vi "TestInsertIntoPanel_OK.vi"(8 "error in (no error)":errorcluster, 11 "TestCase in":refnum<class "TestProtectedSubpanel.lvclass">) -> (0 "error out":errorcluster, 3 "TestCase out":refnum<class "TestProtectedSubpanel.lvclass">)   [LabVIEW 2015, in "TestProtectedSubpanel.lvclass"]
uses:
  TestProtectedSubpanel.lvclass
  ProtectedSubpanel.lvclass
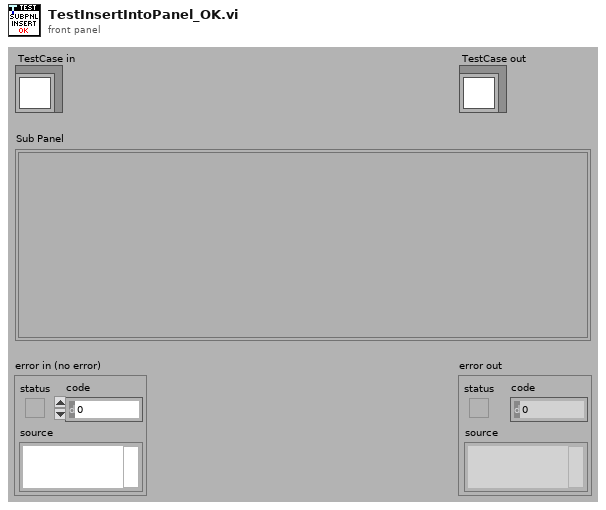
[diagram p1: front panel]
types:
  T1 = typedef "ProtectedSubpanel.lvlib/ProtectedSubpanel.lvclass/Protected Subpanel Reference.ctl" = refnum<data-value>
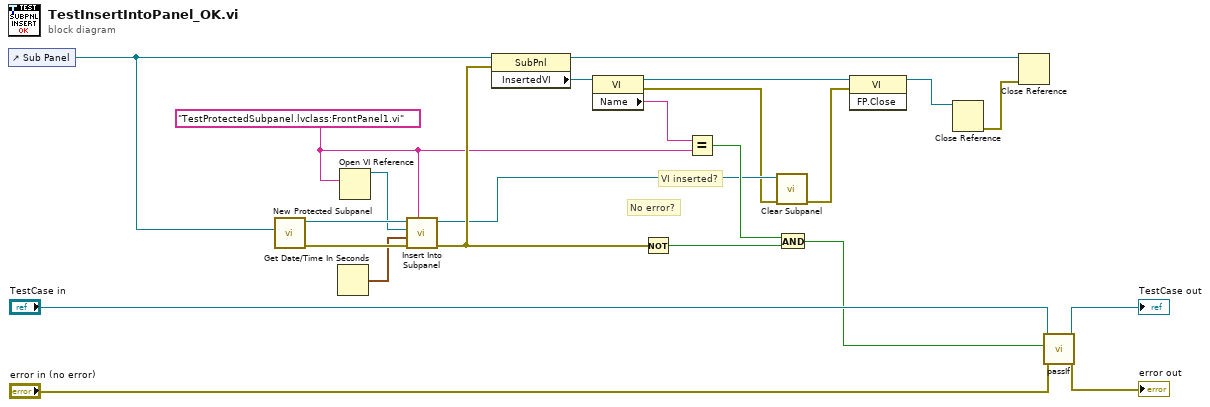
[diagram p0: block diagram]
diagram:
  w11 = "TestProtectedSubpanel.lvclass:FrontPanel1.vi"
  # "No error?"
  # "VI inserted?"
  n1 = control-ref of="Sub Panel"() -> (w17:refnum<vi>)
  n2 = call "New Protected Subpanel.vi"("SubPnl Refnum"=w17) -> ("error out"=w2:errorcluster, "Protected Subpanel"=w19:T1)  [unwired: 9 in]
  n3 = Get Date/Time In Seconds() -> (seconds since 1Jan1904=w1:timestamp)
  n4 = Open VI Reference(vi path=w11) -> (vi reference=w18:refnum<vi>)  [unwired: 5 in, 1 out]
  n5 = call "Insert Into Subpanel.vi"("Viewable Name"=w11, "error in (no error)"=w2, "Insertion Request Time"=w1, "VI Refnum"=w18, "Protected Subpanel"=w19) -> ("error out"=w14:errorcluster, "Protected Subpanel"=w5:T1)  [unwired: 5 in]
  n6 = property class="SubPnl"(reference=w17, error in=w14) -> (reference out=w9:refnum<vi>, "InsertedVI"=w13:refnum<vi>)  [unwired: 1 out]
  n7 = property class="VI"(reference=w13) -> (reference out=w8:refnum<vi>, error out=w3:errorcluster, "Name"=w12:string)  [unwired: 1 in]
  n8 = Not(x=w14) -> (.not. x?=w16:bool)
  n9 = Equal?(x=w12, y=w11) -> (x = y?=w10:bool)
  n10 = call "Clear Subpanel.vi"("error in (no error)"=w3, "Protected Subpanel"=w5) -> ("error out"=w4:errorcluster)  [unwired: 8 in, 1 out]
  n11 = And(x=w10, y=w16) -> (x .and. y?=w15:bool)
  n12 = invoke class="VI" method="FP.Close"(reference=w8, error in=w4) -> (reference out=w6:refnum<vi>)  [unwired: 1 in, 2 out]
  n13 = Close Reference(reference=w6) -> (error out=w7:errorcluster)  [unwired: 1 in]
  n14 = Close Reference(reference=w9, error in (no error)=w7) -> ()  [unwired: 1 out]
  n15 = call-dynamic "passIf.vi"("error in (no error)"="error in (no error)", "pass"=w15, "TestCase in"="TestCase in") -> ("error out"=→"error out":errorcluster, "TestCase out"=→"TestCase out":refnum<class "TestProtectedSubpanel.lvclass">)  [unwired: 7 in]
